vi "Read Offline Data.vi"(8 "Error In":errorcluster) -> (0 "Error Out":errorcluster)   [LabVIEW 2014, in "Aquisicao de Dados.lvlib"]
uses:
  Aquisicao de Dados.lvlib
  <vilib>/Waveform/WDTOps.llb/WDT Waveform Duration DBL.vi
  <vilib>/Waveform/WDTOps.llb/WDT Number of Waveform Samples DBL.vi
  <vilib>/measure/mascope.llb/Amplitude and Levels 1 chan.vi
  <vilib>/express/express analysis/Spectral/Block/exnSpectralBlock spectral measurements peak poly.vi
  <vilib>/express/express analysis/Spectral/Block/exnSpectralBlock spectral measurements peak WFM.vi
  <vilib>/express/express analysis/Spectral/Block/exnSpectralBlock spectral measurements power poly.vi
  <vilib>/express/express analysis/Spectral/Block/exnSpectralBlock spectral measurements power WFM.vi
  <vilib>/express/express analysis/Spectral/XNode/ExpressSpectralMeasurementsBlockNode.xnode
  <vilib>/measure/NI_MAPro.lvlib
panel:
  in  "?":string
  in  "?":string
  in  "Tab Control":enum32{""}(tab)
  in  "?":string
  out "Espectro de Potência":cluster{"f0":dbl, "df":dbl, "magnitude":dbl[]}(graph)
  in  "?":string
  out "Mulher":bool
  out "Frequência \nFundamental":dbl
  out "Homem":bool
  in  "?":string
  out "Canal 1":waveform(dbl)(graph)
  out "Amplitude do Sinal (%) 2":dbl
  out "Número Amostral 2":dbl
  out "Frequência Amostral (Hz) 2":dbl
  out "Período Amostral (s) 2":dbl
  out "Maior Amplitude 2":dbl
  out "Frequência Associada 2":dbl
  out "Resolução de Frequência 2":dbl
  out "Espectro do Canal 1":cluster{"f0":dbl, "df":dbl, "magnitude":dbl[]}(graph)
  out "Espectro do Canal 0":cluster{"f0":dbl, "df":dbl, "magnitude":dbl[]}(graph)
  out "Amplitude do Sinal (%)":dbl
  out "Número Amostral":dbl
  out "Frequência Amostral (Hz)":dbl
  out "Período Amostral (s)":dbl
  out "Maior Amplitude":dbl
  out "Frequência Associada":dbl
  out "Resolução de Frequência":dbl
  out "Canal 0":waveform(dbl)(graph)
  out "Valor de Pico":dbl
  out "Frequência \nde Pico":dbl
  out "Homem":bool
  out "Mulher":bool
  # "Dados do Sinal do Canal 0"
  # "Dados do Sinal do Canal 1"
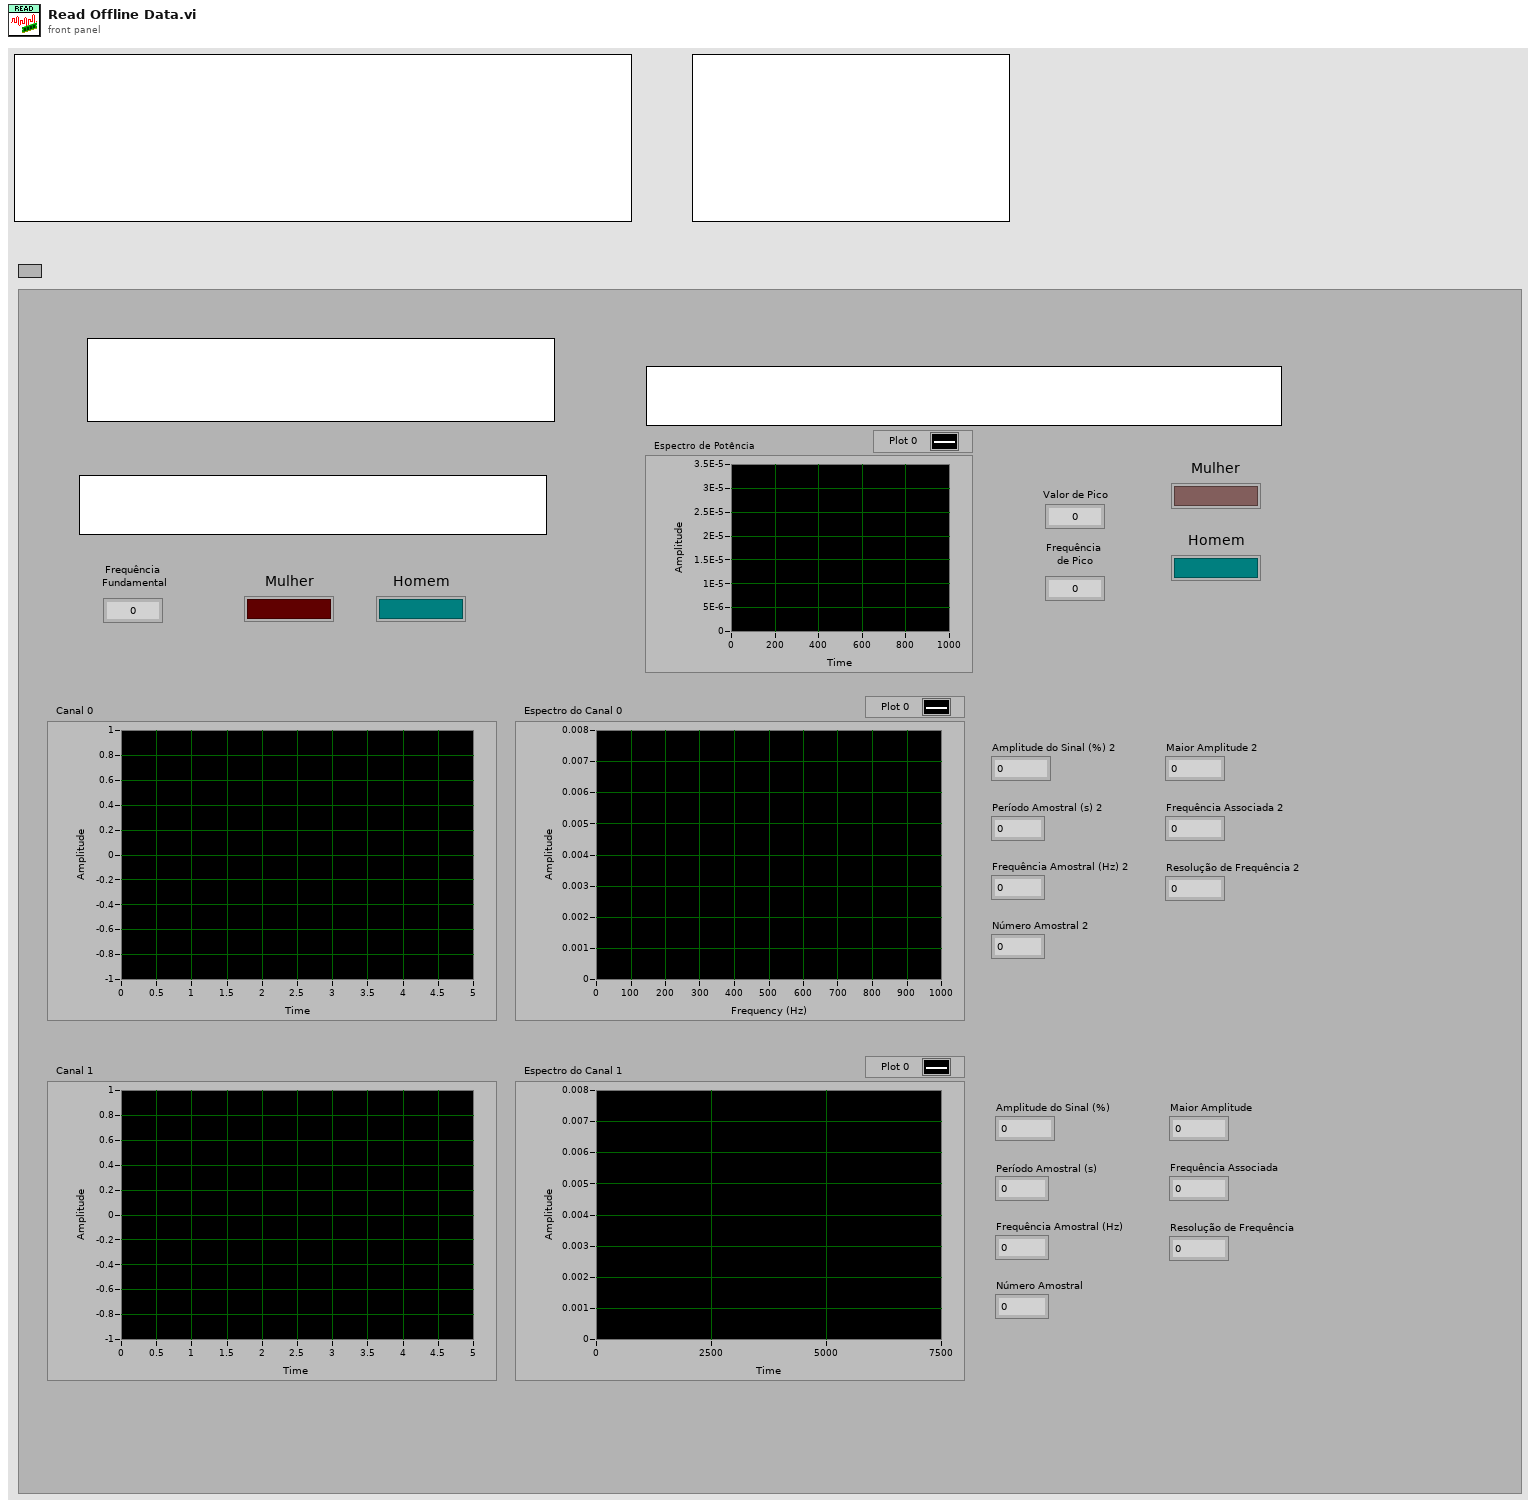
[diagram p1: front panel]
types:
  T1 = enum32{".WAV File", "LTSpice Simulation", "Microphone", "MultiSim Simulation", "Serial Port"}
  T2 = typedef "Aquisicao de Dados.lvlib/_ACC_DATA_ Config DAta State.ctl" = cluster{"_RAW_ Traces":cluster{"Trace Name":string, "Trace Type":string, "Trace Raw Data":dbl[], "Trace Waveform":waveform(dbl)}[], "_WAV_ Traces":waveform(dbl)[], "_MIC_ Config":cluster{"task ID":T3, "Data Chunk Size":i32, "Num Channels":i32, "Resolution":i32, "Sampling Frequency":dbl, "device ID":u32, "Num Chunks":i32}, "_LVM_ Traces":cluster{"Trace Name":string, "Trace Type":string, "Trace Raw Data":dbl[], "Trace Waveform":waveform(dbl)}[]}
  T3 = typedef "Sound Input Task ID.ctl" = u32
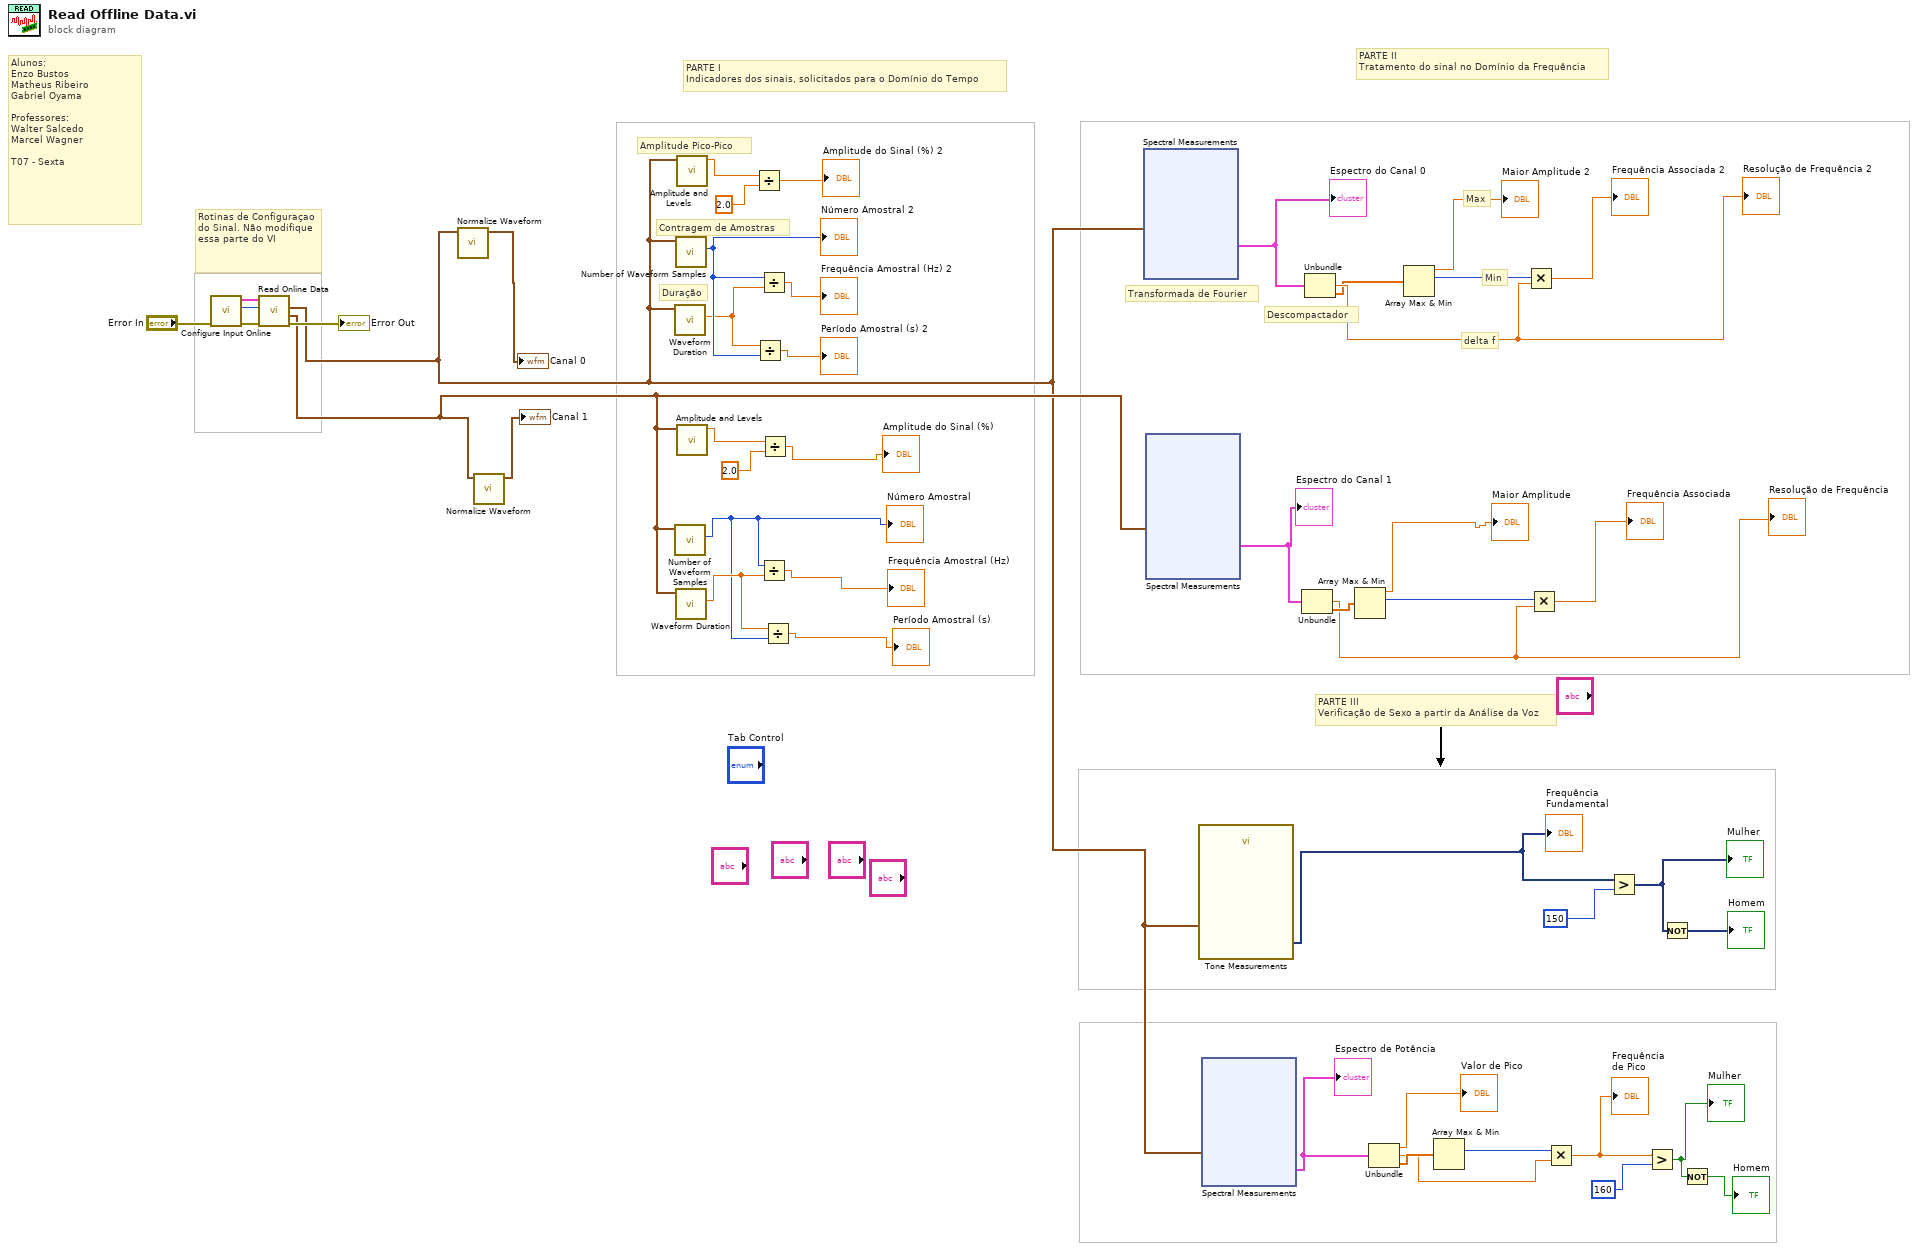
[diagram p0: block diagram]
diagram:
  # "PARTE III\nVerificação de Sexo a partir da Análise da Voz"
  # "Alunos:\nEnzo Bustos\nMatheus Ribeiro\nGabriel Oyama\n\nProfessores:\nWalter Salcedo\nMarcel Wagner\n\nT07 - Sexta"
  # "delta f"
  # "Min"
  # "Max"
  # "Descompactador"
  # "Transformada de Fourier"
  # "Duração"
  # "Contragem de Amostras"
  # "Amplitude Pico-Pico"
  # "PARTE II\nTratamento do sinal no Domínio da Frequência"
  # "PARTE I\nIndicadores dos sinais, solicitados para o Domínio do Tempo"
  # "Rotinas de Configuraçao do Sinal. Não modifique essa parte do VI"
  n1 = call "Configure Input Online.vi"("Error In"="Error In") -> ("Error Out"=w48:errorcluster, "Metodo de Entrada"=w46:T1, "Config Out"=w44:T2)  [unwired: 8 in]
  n2 = call "Read Online Data.vi"("Error In"=w48, "Metodo de Entrada"=w46, "Config Out"=w44) -> ("Error Out"=→"Error Out":errorcluster, "Channel 1"=w16:waveform(dbl), "Channel 0"=w10:waveform(dbl))  [unwired: 6 in]
  n3 = call <vilib>:"Normalize Waveform.vi"("waveform in"=w10) -> ("normalized waveform"=→"Canal 0":waveform(dbl))  [unwired: 7 in, 3 out]
  n4 = call <vilib>:"Normalize Waveform.vi"("waveform in"=w16) -> ("normalized waveform"=→"Canal 1":waveform(dbl))  [unwired: 7 in, 3 out]
  n5 = call-poly <vilib>:"Waveform Duration.vi"("waveform in"=w10) -> ("duration"=w37:dbl)  [unwired: 8 in, 2 out]
  n6 = call-poly <vilib>:"Number of Waveform Samples.vi"("waveform in"=w16) -> ("number of samples"=w27:i32)  [unwired: 8 in, 2 out]
  "Número Amostral" <- w27
  n7 = call-poly <vilib>:"Number of Waveform Samples.vi"("waveform in"=w10) -> ("number of samples"=w38:i32)  [unwired: 8 in, 2 out]
  "Número Amostral 2" <- w38
  n8 = call-poly <vilib>:"Waveform Duration.vi"("waveform in"=w16) -> ("duration"=w34:dbl)  [unwired: 8 in, 2 out]
  n9 = call-poly <vilib>:"Amplitude and Levels.vi"("signal in"=w10) -> ("amplitude"=w42:dbl)  [unwired: 7 in, 3 out]
  n10 = call-poly <vilib>:"Amplitude and Levels.vi"("signal in"=w16) -> ("amplitude"=w40:dbl)  [unwired: 7 in, 3 out]
  n11 = Divide(x=w42, y=2.0) -> (x/y=→"Amplitude do Sinal (%) 2":dbl)
  n12 = Divide(x=w37, y=w38) -> (x/y=→"Período Amostral (s) 2":dbl)
  n13 = Divide(x=w38, y=w37) -> (x/y=→"Frequência Amostral (Hz) 2":dbl)
  n14 = Divide(x=w27, y=w34) -> (x/y=→"Frequência Amostral (Hz)":dbl)
  n15 = Divide(x=w40, y=2.0) -> (x/y=→"Amplitude do Sinal (%)":dbl)
  n16 = Divide(x=w34, y=w27) -> (x/y=→"Período Amostral (s)":dbl)
  n17 = xnode "Spectral Measurements"("Signals"=w10) -> ("FFT - (Peak)"=w14:cluster{"f0":dbl, "df":dbl, "magnitude":dbl[]})  [unwired: 1 in, 2 out]
  "Espectro do Canal 0" <- w14
  n18 = xnode "Spectral Measurements"("Signals"=w16) -> ("FFT - (Peak)"=w31:cluster{"f0":dbl, "df":dbl, "magnitude":dbl[]})  [unwired: 1 in, 2 out]
  "Espectro do Canal 1" <- w31
  n19 = call "Tone Measurements"("Signals"=w10) -> ("Frequency"=w11:dynamicdata)  [unwired: 9 in, 1 out]
  "Frequência \nFundamental" <- w11
  n20 = xnode "Spectral Measurements"("Signals"=w10) -> ("Power Spectrum"=w3:cluster{"f0":dbl, "df":dbl, "magnitude":dbl[]})  [unwired: 1 in, 1 out]
  "Espectro de Potência" <- w3
  n21 = Unbundle(w31) -> ("df"=w24:dbl, "magnitude"=w30:dbl[])  [unwired: 1 out]
  "Resolução de Frequência" <- w24
  n22 = Unbundle(w14) -> ("df"=w29:dbl, "magnitude"=w17:dbl[])  [unwired: 1 out]
  "Resolução de Frequência 2" <- w29
  n23 = Array Max & Min(array=w30) -> (max value=→"Maior Amplitude":dbl, max index (indices)=w32:i32)  [unwired: 2 out]
  n24 = Unbundle(w3) -> ("f0"=→"Valor de Pico":dbl, "df"=w8:dbl, "magnitude"=w9:dbl[])
  n25 = Array Max & Min(array=w17) -> (max value=→"Maior Amplitude 2":dbl, max index (indices)=w33:i32)  [unwired: 2 out]
  n26 = Array Max & Min(array=w9) -> (max index (indices)=w7:i32)  [unwired: 3 out]
  n27 = Multiply(x=w33, y=w29) -> (x*y=→"Frequência Associada 2":dbl)
  n28 = Multiply(x=w32, y=w24) -> (x*y=→"Frequência Associada":dbl)
  n29 = Multiply(x=w7, y=w8) -> (x*y=w5:dbl)
  "Frequência \nde Pico" <- w5
  n30 = Greater?(x=w11, y=150) -> (0:w12:dynamicdata)
  "Mulher" <- w12
  n31 = Greater?(x=w5, y=160) -> (0:w2:bool)
  "Mulher" <- w2
  n32 = Not(x=w12) -> (.not. x?=→"Homem":dynamicdata)
  n33 = Not(x=w2) -> (.not. x?=→"Homem":bool)
